vi "_RT_Pub_FlashRW.vi"(5 "FileEnum":T1(ring), 7 "State":enum16{"Read", "Write"}(ring), 8 "error in (no error)":errorcluster, 10 "DataIn":variant) -> (0 "error out":errorcluster, 2 "Value":variant, 3 "dup path":path)   [LabVIEW 2018]
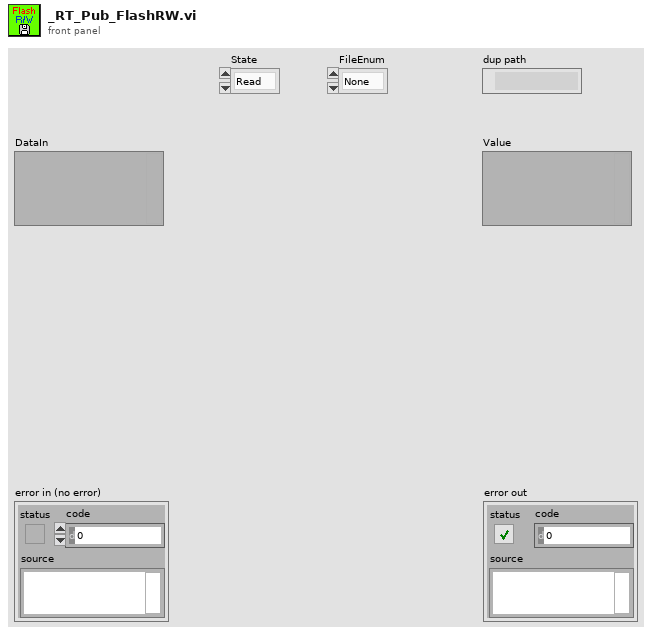
[diagram p1: front panel]
types:
  T1 = enum16{"None", "D999", "ExtAO", "ExtDO", "ExtDI_Label", "Signal_Remarks", "Script"}
  T2 = enum16{"open", "replace", "create", "open or create", "replace or create", "replace or create with confirmation"}
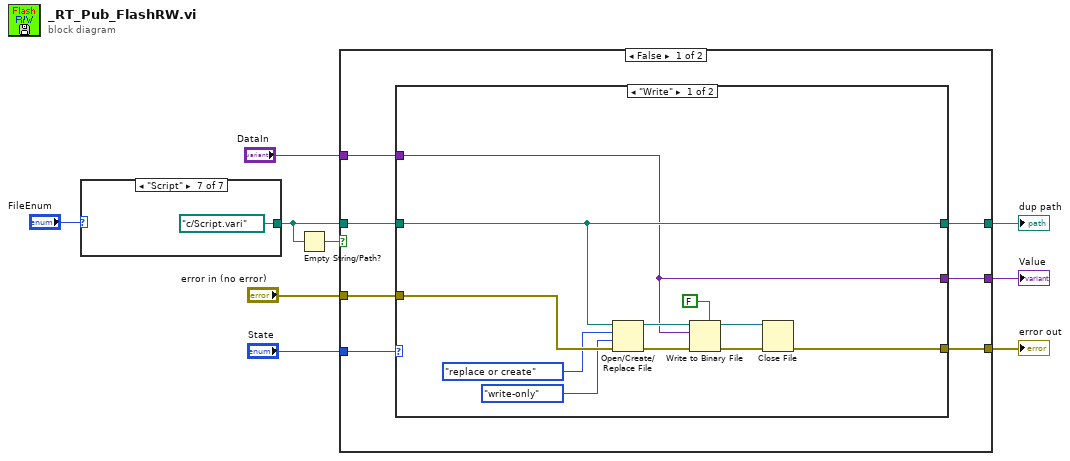
[diagram p0: block diagram]
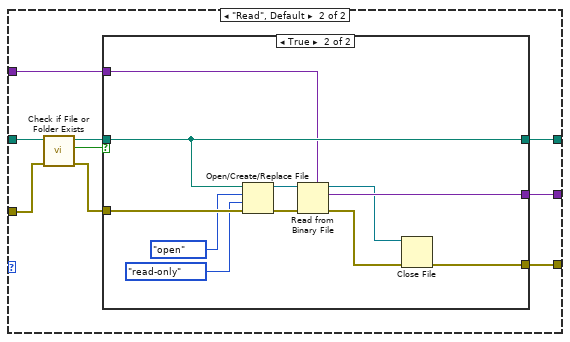
[diagram p2: hidden frame]
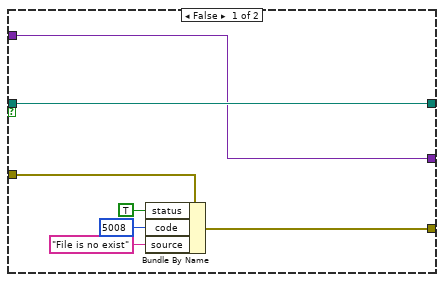
[diagram p3: hidden frame]
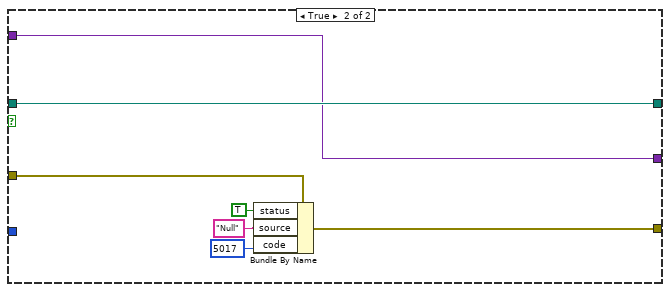
[diagram p4: hidden frame]
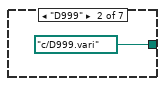
[diagram p6: hidden frame]
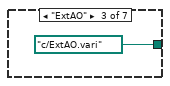
[diagram p7: hidden frame]
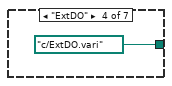
[diagram p8: hidden frame]
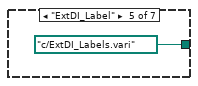
[diagram p9: hidden frame]
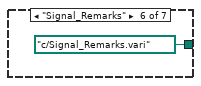
[diagram p10: hidden frame]
diagram:
  n1 = case shown="\"Script\"" "FileEnum" {
    tunnel: [_ path "c:/D999.vari" ("file path (use dialog)") path "c:/ExtAO.vari" ("file path (use dialog)") path "c:/ExtDO.vari" ("file path (use dialog)") path "c:/ExtDI_Labels.vari" ("file path (use dialog)") path "c:/Signal_Remarks.vari" ("file path (use dialog)") path "c:/Script.vari" ("file path (use dialog)")] -> w2
    frame "None", Default {
    }
    frame "D999" {
    }
    frame "ExtAO" {
    }
    frame "ExtDO" {
    }
    frame "ExtDI_Label" {
    }
    frame "Signal_Remarks" {
    }
    frame "Script" {
    }
  }
  n2 = Empty String/Path?(string/path=w2) -> (empty?=w3:bool)
  n3 = case shown="False" w3 {
    tunnel: [w22 w67] -> w9
    tunnel: [w21 w61] -> w1
    tunnel: "error in (no error)" -> [w20 w62]
    tunnel: "State" -> [w19 _]
    tunnel: "DataIn" -> [w18 w66]
    tunnel: [w17 w66] -> w4
    tunnel: w2 -> [w16 w67]
    frame False {
      n4 = case shown="\"Write\"" w19 {
        tunnel: [w29 w39] -> w22
        tunnel: [w28 w38] -> w21
        tunnel: w20 -> [w33 w37]
        tunnel: w16 -> [w29 w36]
        tunnel: w18 -> [w23 w35]
        tunnel: [w23 w34] -> w17
        frame "Write" {
          n5 = Open/Create/Replace File(file path (use dialog)=w29, error in=w33, operation (0:open)=T2."replace or create", access (0:read/write)=enum16{"read/write", "read-only", "write-only"}."write-only") -> (refnum out=w31:refnum<file>, error out=w30:errorcluster)  [unwired: 2 in, 1 out]
          n6 = Write to Binary File(file (use dialog)=w31, data=w23, error in=w30, 5:FALSE ("prepend array or string size? (T)")) -> (refnum out=w26:refnum<file>, error out=w27:errorcluster)  [unwired: 2 in, 1 out]
          n7 = Close File(refnum=w26, error in=w27) -> (error out=w28:errorcluster)  [unwired: 1 out]
        }
        frame "Read", Default {
          n8 = call <vilib>:"Check if File or Folder Exists.vi"("error in (no error)"=w37, "path"=w36) -> ("error out"=w40:errorcluster, "file or folder exists?"=w42:bool, "dup path"=w41:path)  [unwired: 7 in]
          n9 = case shown="True" w42 {
            tunnel: w41 -> [w49 w59]
            tunnel: w40 -> [w47 w60]
            tunnel: [w49 w59] -> w39
            tunnel: [w48 w56] -> w34
            tunnel: [w43 w50] -> w38
            tunnel: w35 -> [w48 w53]
            frame False {
              n10 = Bundle By Name(cluster=w47, "status"=TRUE, "code"=5008, "source"="File is no exist") -> (w43:errorcluster)
            }
            frame True {
              n11 = Open/Create/Replace File(file path (use dialog)=w59, error in=w60, operation (0:open)=T2."open", access (0:read/write)=enum16{"read/write", "read-only", "write-only"}."read-only") -> (refnum out=w58:refnum<file>, error out=w57:errorcluster)  [unwired: 2 in, 1 out]
              n12 = Read from Binary File(5:w53, 8:w57, 11:w58) -> (0:w54:errorcluster, 2:w56:variant, 3:w55:refnum<file>)  [unwired: 3 in, 1 out]
              n13 = Close File(refnum=w55, error in=w54) -> (error out=w50:errorcluster)  [unwired: 1 out]
            }
          }
        }
      }
    }
    frame True {
      n14 = Bundle By Name(cluster=w62, "status"=TRUE, "source"="Null", "code"=5017) -> (w61:errorcluster)
    }
  }
  "dup path" <- w9
  "error out" <- w1
  "Value" <- w4
